vi "port_multiple_target.vi"(3 "LV Version":string, 4 "OS Specific path":T1(array[cluster]), 5 "Generated ini location path":string="C:\\Weekly Runs\\Generated ini\\", 6 "Target File Path":path, 7 "General INI path":path, 8 "error in":errorcluster, 9 "Bitness":string, 10 "VM Name":string, 11 "Listbox  Target":i32[](listbox)) -> (0 "error out":errorcluster)   [LabVIEW 2015]
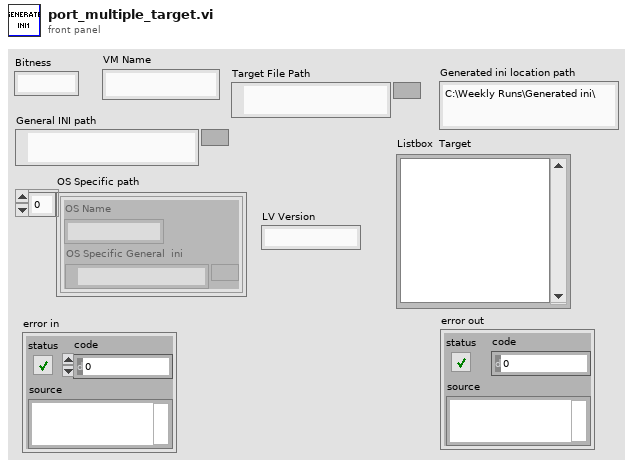
[diagram p1: front panel]
types:
  T1 = cluster{"OS Name":string, "OS Specific General  ini":path}[]
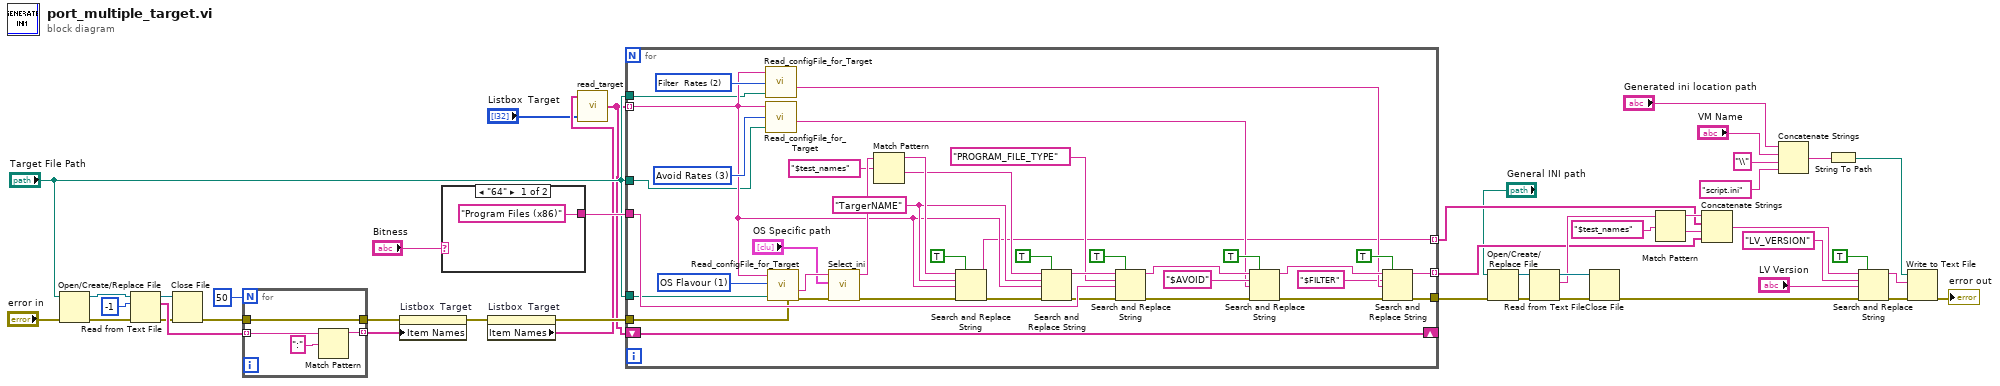
[diagram p0: block diagram]
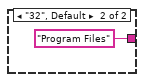
[diagram p2: hidden frame]
diagram:
  n1 = Open/Create/Replace File(file path (use dialog)="Target File Path", error in="error in") -> (refnum out=w38:refnum<file>, error out=w39:errorcluster)  [unwired: 4 in, 1 out]
  n2 = Read from Text File(file (use dialog)=w38, count=-1, error in=w39) -> (refnum out=w45:refnum<file>, text=w43:string[], error out=w40:errorcluster)  [unwired: 1 in, 1 out]
  n3 = Close File(refnum=w45, error in=w40) -> (error out=w41:errorcluster)  [unwired: 1 out]
  n4 = for {
    N: 50 -> [_]
    tunnel: [w49] -> w12 mode=indexing
    tunnel: [w48] -> w14
    tunnel: w41 -> [w48]
    tunnel: w43 -> [w46] mode=indexing
    n5 = Match Pattern(string=w46, regular expression=":") -> (before substring=w49:string)  [unwired: 1 in, 3 out]
  }
  n6 = property on="Listbox  Target" class="LstBox (strict)"(error in=w14, "Item Names"=w12) -> (error out=w13:errorcluster)  [unwired: 1 in, 1 out]
  n7 = case shown="\"64\"" "Bitness" {
    tunnel: ["Program Files (x86)" ("search string/char (-)") "Program Files" ("search string/char (-)")] -> w23
    frame "64" {
    }
    frame "32", Default {
    }
  }
  n8 = property on="Listbox  Target" class="LstBox (strict)"(error in=w13) -> (error out=w11:errorcluster, "Item Names"=w10:string[])  [unwired: 1 in, 1 out]
  n9 = call "read_target.vi"("Listbox  Target"="Listbox  Target", "Item Names"=w10) -> ("Array"=w8:string[])
  n10 = for {
    tunnel: w8 -> [w66] mode=indexing
    tunnel: w23 -> [w79]
    shift-right: [w68] -> _
    shift-left: w8 -> [w68]
    tunnel: [w52] -> w22 mode=indexing
    tunnel: [w54] -> w19 mode=indexing
    tunnel: w11 -> [w58]
    tunnel: [w55] -> w17
    tunnel: "Target File Path" -> [w62]
    tunnel: "Target File Path" -> [w61]
    tunnel: "Target File Path" -> [w60]
    w82 = "TargerNAME" ("search string/char (-)")
    w88 = u16 2 items=["Target Nmae", "OS Flavour", "Filter  Rates", "Avoid Rates"] ("Ring 2")
    w89 = u16 3 items=["Target Nmae", "OS Flavour", "Filter  Rates", "Avoid Rates"] ("Ring 2")
    w90 = u16 1 items=["Target Nmae", "OS Flavour", "Filter  Rates", "Avoid Rates"] ("Ring 2")
    n11 = call "Read_configFile_for_Target.vi"("Target File Path"=w62, "Ring 2"=w88, "Target Name"=w66) -> ("selected target"=w70:string)  [unwired: 4 in, 1 out]
    n12 = call "Read_configFile_for_Target.vi"("Target File Path"=w61, "Ring 2"=w89, "Target Name"=w66) -> ("selected target"=w71:string)  [unwired: 4 in, 1 out]
    n13 = call "Read_configFile_for_Target.vi"("error in"=w58, "Target File Path"=w60, "Ring 2"=w90, "Target Name"=w66) -> ("error out"=w59:errorcluster, "selected target"=w67:string)  [unwired: 3 in]
    n14 = call "Select_ini.vi"("error in"=w59, "OS Specific path"="OS Specific path", "OS Name"=w67) -> ("error out"=w57:errorcluster, "OS Apecific INI"=w87:string)  [unwired: 7 in]
    n15 = Match Pattern(string=w87, regular expression="$test_names" ("search string/char (-)")) -> (before substring=w85:string, after substring=w83:string)  [unwired: 1 in, 2 out]
    n16 = Search and Replace String(replace all?=TRUE ("replace all? (F)"), input string=w85, search string=w82, replace string=w66, error in=w57) -> (result string=w52:string, error out=w53:errorcluster)  [unwired: 3 in, 2 out]
    n17 = Search and Replace String(replace all?=TRUE ("replace all? (F)"), input string=w83, search string=w82, replace string=w66, error in=w53) -> (result string=w81:string, error out=w65:errorcluster)  [unwired: 3 in, 2 out]
    n18 = Search and Replace String(replace all?=TRUE ("replace all? (F)"), input string=w81, search string="PROGRAM_FILE_TYPE" ("search string/char (-)"), replace string=w79, error in=w65) -> (result string=w74:string, error out=w64:errorcluster)  [unwired: 3 in, 2 out]
    n19 = Search and Replace String(replace all?=TRUE ("replace all? (F)"), input string=w74, search string="$AVOID" ("search string/char (-)"), replace string=w71, error in=w64) -> (result string=w73:string, error out=w63:errorcluster)  [unwired: 3 in, 2 out]
    n20 = Search and Replace String(replace all?=TRUE ("replace all? (F)"), input string=w73, search string="$FILTER" ("search string/char (-)"), replace string=w70, error in=w63) -> (result string=w54:string, error out=w55:errorcluster)  [unwired: 3 in, 2 out]
  }
  n21 = Open/Create/Replace File(file path (use dialog)="General INI path", error in=w17) -> (refnum out=w35:refnum<file>, error out=w36:errorcluster)  [unwired: 4 in, 1 out]
  n22 = Read from Text File(file (use dialog)=w35, error in=w36) -> (refnum out=w33:refnum<file>, text=w32:string, error out=w34:errorcluster)  [unwired: 2 in, 1 out]
  n23 = Close File(refnum=w33, error in=w34) -> (error out=w6:errorcluster)  [unwired: 1 out]
  n24 = Match Pattern(string=w32, regular expression="$test_names" ("search string/char (-)")) -> (before substring=w30:string, after substring=w20:string)  [unwired: 1 in, 2 out]
  n25 = Concatenate Strings(w30, w22, w20, w19) -> (w7:string)
  n26 = Concatenate Strings("Generated ini location path", "VM Name", "\\", "script.ini") -> (w28:string)
  n27 = String To Path(string=w28) -> (path=w25:path)
  n28 = Search and Replace String(replace all?=TRUE ("replace all? (F)"), input string=w7, search string="LV_VERSION", replace string="LV Version", error in=w6) -> (result string=w4:string, error out=w5:errorcluster)  [unwired: 3 in, 2 out]
  n29 = Write to Text File(file (use dialog)=w25, text=w4, error in=w5) -> (error out=→"error out":errorcluster)  [unwired: 1 in, 2 out]
